vi "CCE RRMA P03 SubVI01.vi"(10 "CAPA DE COLOR":T2(ring)=enum."RGB2GRAY MATLAB", 11 "Image":T1) -> (3 "Array":u8[][](array[numeric]))   [LabVIEW 2020]
doc: "Ceballos Conde Emanuel Rodríguez Ramírez Miguel Ángel 4MV6 Sistemas de visión artificial 2022/1\neste vi permite hacer la conversion obtener una capa de las componentes RGB, HSV,CMY o escala de grisis,"
uses:
  <vilib>/vision/Image Controls.llb/IMAQ Image.ctl
panel:
  # "Ceballos Conde Emanuel\nRodríguez Ramírez Miguel Ángel\n4MV6\nSistemas de visión artificial\n2022/1"
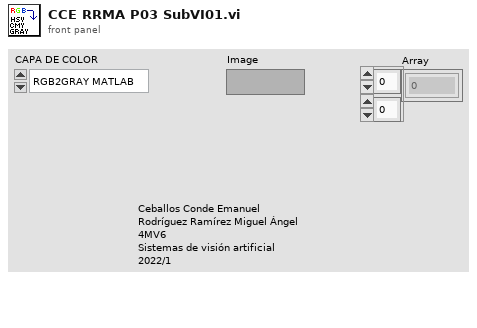
[diagram p1: front panel]
types:
  T1 = typedef "IMAQ Image.ctl" = refnum<image>
  T2 = enum16{"H", "S", "V", "C", "M", "Y", "R", "G", "B", "RGB2GRAY MATLAB"}
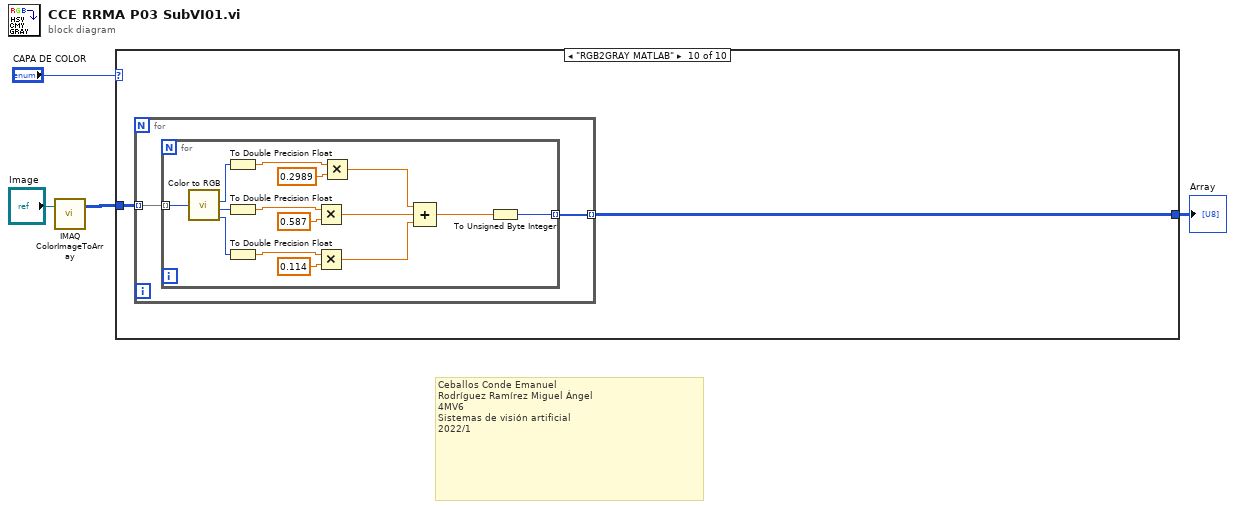
[diagram p0: block diagram]
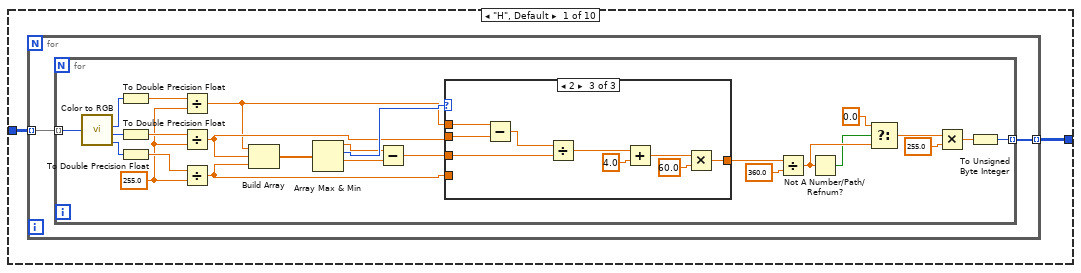
[diagram p2: hidden frame]
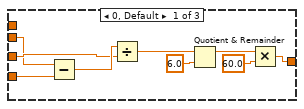
[diagram p3: hidden frame]
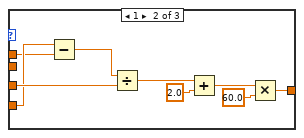
[diagram p4: hidden frame]
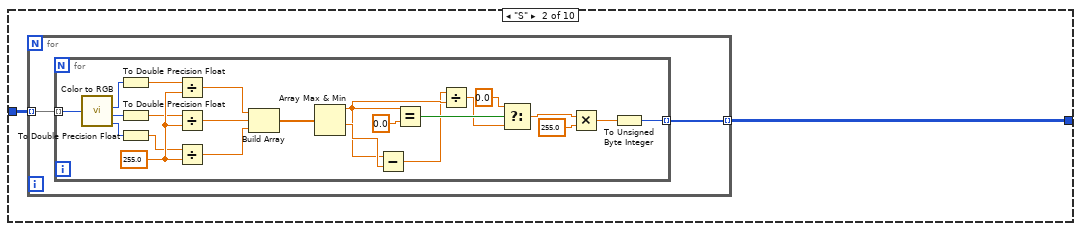
[diagram p5: hidden frame]
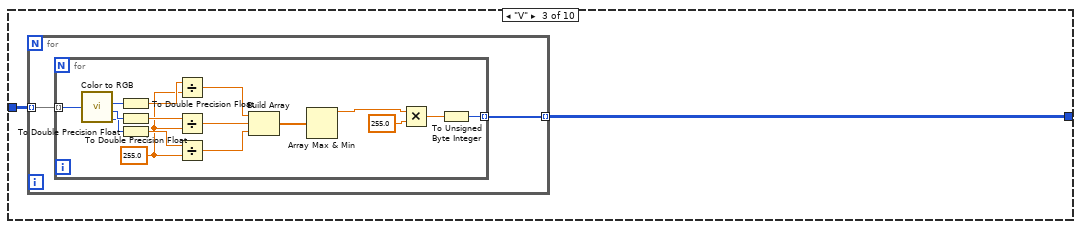
[diagram p6: hidden frame]
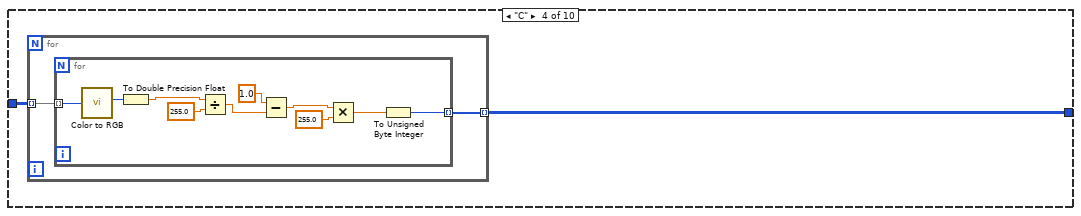
[diagram p7: hidden frame]
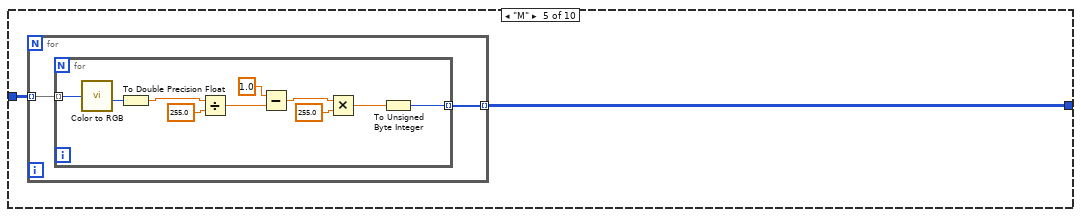
[diagram p8: hidden frame]
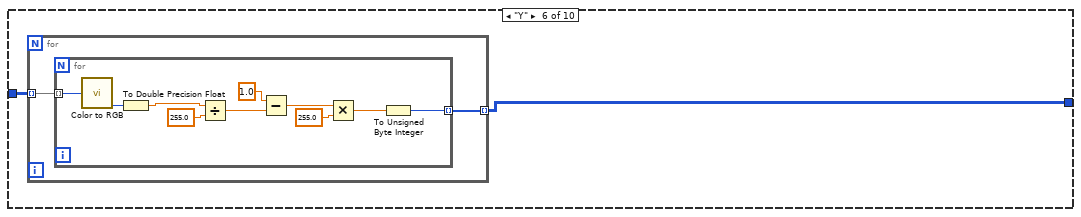
[diagram p9: hidden frame]
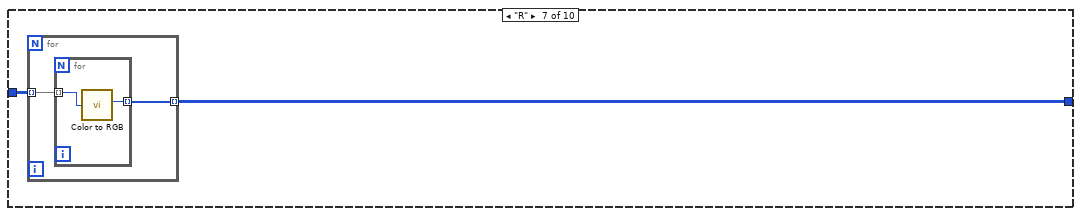
[diagram p10: hidden frame]
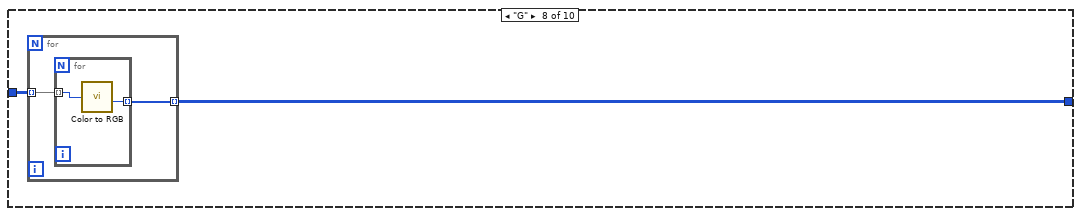
[diagram p11: hidden frame]
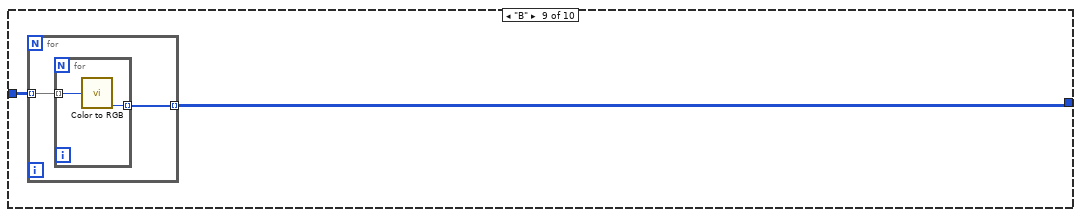
[diagram p12: hidden frame]
diagram:
  # "Ceballos Conde Emanuel\nRodríguez Ramírez Miguel Ángel\n4MV6\nSistemas de visión artificial\n2022/1"
  n1 = call "IMAQ ColorImageToArray"("Image"="Image") -> ("Image Pixels (U32)"=w3:u32[][])  [unwired: 3 in, 2 out]
  n2 = case shown="\"RGB2GRAY MATLAB\"" "CAPA DE COLOR" {
    tunnel: [w6 w62 w89 w108 w122 w136 w150 w156 w162 w168] -> w2
    tunnel: w3 -> [w5 w61 w88 w109 w123 w137 w151 w157 w163 w169]
    frame "H", Default {
      n3 = for {
        tunnel: [w8] -> w6 mode=indexing
        tunnel: w5 -> [w7] mode=indexing
        n4 = for {
          tunnel: [w9] -> w8 mode=indexing
          tunnel: w7 -> [w16] mode=indexing
          w19 = 255.0 ("y")
          n5 = call <vilib>:"Color to RGB.vi"("Color"=w16) -> ("R"=w15:u8, "G"=w14:u8, "B"=w13:u8)  [unwired: 1 out]
          n6 = To Double Precision Float(number=w15) -> (double precision float=w20:dbl)
          n7 = To Double Precision Float(number=w14) -> (double precision float=w21:dbl)
          n8 = To Double Precision Float(number=w13) -> (double precision float=w22:dbl)
          n9 = Divide(x=w20, y=w19) -> (x/y=w28:dbl)
          n10 = Divide(x=w21, y=w19) -> (x/y=w29:dbl)
          n11 = Divide(x=w22, y=w19) -> (x/y=w30:dbl)
          n12 = Build Array(w28, w29, w30) -> (w23:dbl[])
          n13 = Array Max & Min(array=w23) -> (max value=w25:dbl, max index (indices)=w33:i32, min value=w24:dbl)  [unwired: 1 out]
          n14 = Subtract(x=w25, y=w24) -> (x-y=w26:dbl)
          n15 = case shown="2" w33 {
            tunnel: [w36 w45 w54] -> w27
            tunnel: w29 -> [w35 _ w52]
            tunnel: w30 -> [w34 w44 _]
            tunnel: w26 -> [w41 w50 w59]
            tunnel: w28 -> [_ w43 w53]
            frame 0, Default {
              n16 = Subtract(x=w35, y=w34) -> (x-y=w42:dbl)
              n17 = Divide(x=w42, y=w41) -> (x/y=w40:dbl)
              n18 = Quotient & Remainder(x=w40, y=6.0) -> (x-y*floor(x/y)=w37:dbl)  [unwired: 1 out]
              n19 = Multiply(x=w37, y=60.0) -> (x*y=w36:dbl)
            }
            frame 1 {
              n20 = Subtract(x=w44, y=w43) -> (x-y=w51:dbl)
              n21 = Divide(x=w51, y=w50) -> (x/y=w49:dbl)
              n22 = Add(x=w49, y=2.0) -> (x+y=w46:dbl)
              n23 = Multiply(x=w46, y=60.0) -> (x*y=w45:dbl)
            }
            frame 2 {
              n24 = Subtract(x=w53, y=w52) -> (x-y=w60:dbl)
              n25 = Divide(x=w60, y=w59) -> (x/y=w58:dbl)
              n26 = Add(x=w58, y=4.0) -> (x+y=w55:dbl)
              n27 = Multiply(x=w55, y=60.0) -> (x*y=w54:dbl)
            }
          }
          n28 = Divide(x=w27, y=360.0) -> (x/y=w32:dbl)
          n29 = Not A Number/Path/Refnum?(number/path/refnum=w32) -> (NaN/Path/Refnum?=w31:bool)
          n30 = Select(t=0.0, s=w31, f=w32) -> (s? t:f=w11:dbl)
          n31 = Multiply(x=w11, y=255.0) -> (x*y=w12:dbl)
          n32 = To Unsigned Byte Integer(number=w12) -> (unsigned 8bit integer=w9:u8)
        }
      }
    }
    frame "S" {
      n33 = for {
        tunnel: [w64] -> w62 mode=indexing
        tunnel: w61 -> [w63] mode=indexing
        n34 = for {
          tunnel: [w65] -> w64 mode=indexing
          tunnel: w63 -> [w72] mode=indexing
          w87 = 255.0 ("y")
          n35 = call <vilib>:"Color to RGB.vi"("Color"=w72) -> ("R"=w71:u8, "G"=w70:u8, "B"=w69:u8)  [unwired: 1 out]
          n36 = To Double Precision Float(number=w71) -> (double precision float=w86:dbl)
          n37 = To Double Precision Float(number=w70) -> (double precision float=w85:dbl)
          n38 = To Double Precision Float(number=w69) -> (double precision float=w84:dbl)
          n39 = Divide(x=w86, y=w87) -> (x/y=w75:dbl)
          n40 = Divide(x=w85, y=w87) -> (x/y=w74:dbl)
          n41 = Divide(x=w84, y=w87) -> (x/y=w73:dbl)
          n42 = Build Array(w75, w74, w73) -> (w83:dbl[])
          n43 = Array Max & Min(array=w83) -> (max value=w77:dbl, min value=w79:dbl)  [unwired: 2 out]
          n44 = Subtract(x=w77, y=w79) -> (x-y=w76:dbl)
          n45 = Equal?(x=w77, y=0.0) -> (x = y?=w81:bool)
          n46 = Divide(x=w76, y=w77) -> (x/y=w78:dbl)
          n47 = Select(t=0.0, s=w81, f=w78) -> (s? t:f=w67:dbl)
          n48 = Multiply(x=w67, y=255.0) -> (x*y=w66:dbl)
          n49 = To Unsigned Byte Integer(number=w66) -> (unsigned 8bit integer=w65:u8)
        }
      }
    }
    frame "V" {
      n50 = for {
        tunnel: [w91] -> w89 mode=indexing
        tunnel: w88 -> [w90] mode=indexing
        n51 = for {
          tunnel: [w92] -> w91 mode=indexing
          tunnel: w90 -> [w99] mode=indexing
          w101 = 255.0 ("y")
          n52 = call <vilib>:"Color to RGB.vi"("Color"=w99) -> ("R"=w98:u8, "G"=w97:u8, "B"=w96:u8)  [unwired: 1 out]
          n53 = To Double Precision Float(number=w98) -> (double precision float=w102:dbl)
          n54 = To Double Precision Float(number=w97) -> (double precision float=w103:dbl)
          n55 = To Double Precision Float(number=w96) -> (double precision float=w104:dbl)
          n56 = Divide(x=w102, y=w101) -> (x/y=w106:dbl)
          n57 = Divide(x=w103, y=w101) -> (x/y=w100:dbl)
          n58 = Divide(x=w104, y=w101) -> (x/y=w107:dbl)
          n59 = Build Array(w106, w100, w107) -> (w105:dbl[])
          n60 = Array Max & Min(array=w105) -> (max value=w94:dbl)  [unwired: 3 out]
          n61 = Multiply(x=w94, y=255.0) -> (x*y=w93:dbl)
          n62 = To Unsigned Byte Integer(number=w93) -> (unsigned 8bit integer=w92:u8)
        }
      }
    }
    frame "C" {
      n63 = for {
        tunnel: w109 -> [w111] mode=indexing
        tunnel: [w110] -> w108 mode=indexing
        n64 = for {
          tunnel: w111 -> [w121] mode=indexing
          tunnel: [w112] -> w110 mode=indexing
          n65 = call <vilib>:"Color to RGB.vi"("Color"=w121) -> ("R"=w120:u8)  [unwired: 3 out]
          n66 = To Double Precision Float(number=w120) -> (double precision float=w116:dbl)
          n67 = Divide(x=w116, y=255.0) -> (x/y=w118:dbl)
          n68 = Subtract(x=1.0, y=w118) -> (x-y=w115:dbl)
          n69 = Multiply(x=w115, y=255.0) -> (x*y=w113:dbl)
          n70 = To Unsigned Byte Integer(number=w113) -> (unsigned 8bit integer=w112:u8)
        }
      }
    }
    frame "M" {
      n71 = for {
        tunnel: w123 -> [w125] mode=indexing
        tunnel: [w124] -> w122 mode=indexing
        n72 = for {
          tunnel: w125 -> [w135] mode=indexing
          tunnel: [w127] -> w124 mode=indexing
          n73 = call <vilib>:"Color to RGB.vi"("Color"=w135) -> ("G"=w126:u8)  [unwired: 3 out]
          n74 = To Double Precision Float(number=w126) -> (double precision float=w131:dbl)
          n75 = Divide(x=w131, y=255.0) -> (x/y=w133:dbl)
          n76 = Subtract(x=1.0, y=w133) -> (x-y=w130:dbl)
          n77 = Multiply(x=w130, y=255.0) -> (x*y=w128:dbl)
          n78 = To Unsigned Byte Integer(number=w128) -> (unsigned 8bit integer=w127:u8)
        }
      }
    }
    frame "Y" {
      n79 = for {
        tunnel: w137 -> [w139] mode=indexing
        tunnel: [w138] -> w136 mode=indexing
        n80 = for {
          tunnel: w139 -> [w149] mode=indexing
          tunnel: [w141] -> w138 mode=indexing
          n81 = call <vilib>:"Color to RGB.vi"("Color"=w149) -> ("B"=w140:u8)  [unwired: 3 out]
          n82 = To Double Precision Float(number=w140) -> (double precision float=w145:dbl)
          n83 = Divide(x=w145, y=255.0) -> (x/y=w147:dbl)
          n84 = Subtract(x=1.0, y=w147) -> (x-y=w144:dbl)
          n85 = Multiply(x=w144, y=255.0) -> (x*y=w142:dbl)
          n86 = To Unsigned Byte Integer(number=w142) -> (unsigned 8bit integer=w141:u8)
        }
      }
    }
    frame "R" {
      n87 = for {
        tunnel: w151 -> [w153] mode=indexing
        tunnel: [w152] -> w150 mode=indexing
        n88 = for {
          tunnel: w153 -> [w155] mode=indexing
          tunnel: [w154] -> w152 mode=indexing
          n89 = call <vilib>:"Color to RGB.vi"("Color"=w155) -> ("R"=w154:u8)  [unwired: 3 out]
        }
      }
    }
    frame "G" {
      n90 = for {
        tunnel: w157 -> [w159] mode=indexing
        tunnel: [w158] -> w156 mode=indexing
        n91 = for {
          tunnel: w159 -> [w161] mode=indexing
          tunnel: [w160] -> w158 mode=indexing
          n92 = call <vilib>:"Color to RGB.vi"("Color"=w161) -> ("G"=w160:u8)  [unwired: 3 out]
        }
      }
    }
    frame "B" {
      n93 = for {
        tunnel: w163 -> [w165] mode=indexing
        tunnel: [w164] -> w162 mode=indexing
        n94 = for {
          tunnel: w165 -> [w167] mode=indexing
          tunnel: [w166] -> w164 mode=indexing
          n95 = call <vilib>:"Color to RGB.vi"("Color"=w167) -> ("B"=w166:u8)  [unwired: 3 out]
        }
      }
    }
    frame "RGB2GRAY MATLAB" {
      n96 = for {
        tunnel: w169 -> [w171] mode=indexing
        tunnel: [w170] -> w168 mode=indexing
        n97 = for {
          tunnel: w171 -> [w186] mode=indexing
          tunnel: [w175] -> w170 mode=indexing
          n98 = call <vilib>:"Color to RGB.vi"("Color"=w186) -> ("R"=w185:u8, "G"=w184:u8, "B"=w183:u8)  [unwired: 1 out]
          n99 = To Double Precision Float(number=w185) -> (double precision float=w174:dbl)
          n100 = To Double Precision Float(number=w184) -> (double precision float=w173:dbl)
          n101 = To Double Precision Float(number=w183) -> (double precision float=w172:dbl)
          n102 = Multiply(x=w173, y=0.587) -> (x*y=w178:dbl)
          n103 = Multiply(x=w172, y=0.114) -> (x*y=w177:dbl)
          n104 = Multiply(x=w174, y=0.2989) -> (x*y=w179:dbl)
          n105 = Compound Arithmetic op=ADD(w179, w178, w177) -> (w176:dbl)
          n106 = To Unsigned Byte Integer(number=w176) -> (unsigned 8bit integer=w175:u8)
        }
      }
    }
  }
  "Array" <- w2
